vi "Read TCPClient.vi"(8 "error in (no error)":errorcluster, 11 "TCPClient in":refnum<class "TCPClient.lvclass">) -> (0 "error out":errorcluster, 2 "tcp.lvlib:TCPClient.lvclass":refnum<class "TCPClient.lvclass">, 3 "TCPClient out":refnum<class "TCPClient.lvclass">)   [LabVIEW 2016, in "TCPClient.lvclass"]
uses:
  TCPClient.lvclass
  common_ascii_tcp/TCPClient/TCPClient.lvclass
  TCPClient.lvclass/TCPClient.ctl
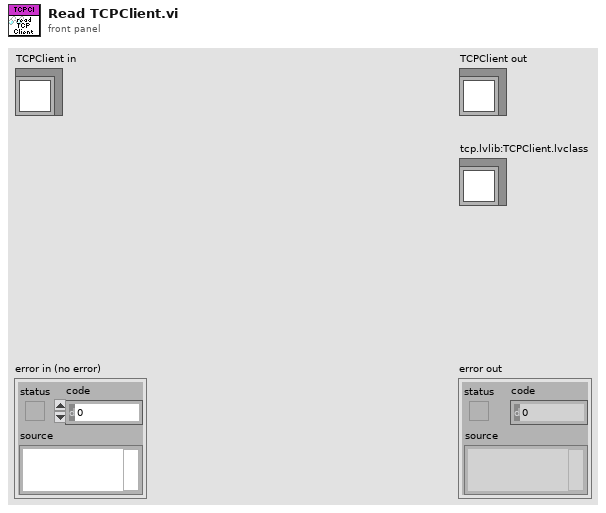
[diagram p1: front panel]
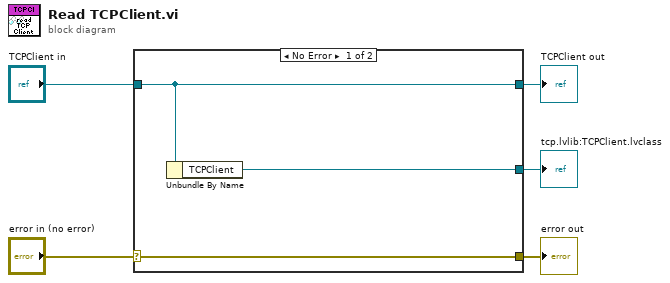
[diagram p0: block diagram]
diagram:
  n1 = case shown="No Error" "error in (no error)" {
    selector: "error in (no error)" -> [w8 w9]
    tunnel: [w8 w9] -> w4
    tunnel: [w7 w10] -> w2
    tunnel: "TCPClient in" -> [w7 w10]
    tunnel: [w6 _] -> w1
    frame No Error {
      n2 = Unbundle By Name(w7) -> ("TCPClient"=w6:refnum<class "TCPClient.lvclass">)
    }
    frame Error {
    }
  }
  "error out" <- w4
  "TCPClient out" <- w2
  "tcp.lvlib:TCPClient.lvclass" <- w1
